vi "Demo.vi"() -> ()   [LabVIEW 2017]
uses:
  Components/ViPER.lvlibp/ViPER.lvclass
panel:
  in  "stop":bool
  out "error out":errorcluster
  in  "Config XML":string="<?xml version=\"1.0\" encoding=\"UTF-8\" standalone=\"no\" ?>\n<Object>\n\n  <Name>panel</Name>\n\n  <Class>DUT_Handler_Bailey_Panel</Class>\n\n  <Config>\n    <NumElts>1</NumElts>\n    <U32>\n      <Name>DUT Quantity</Name>\n      <Val>6</Val>\n</U32>\n</Config>  <Objects>\n    <Object>\n      <Name>Barcode</Name>\n      <Class>QR_Reader_Honeywell_3310G</Class>\n      <Config>\n        <NumElts>1</NumElts>\n        <Refnum>\n          <Name>ComPort</Name>\n          <RefKind>VISA</RefKind>\n          <Val>COM6</Val>\n</Refnum>\n</Config>    </Object>\n  </Objects>\n\n</Object>\n"
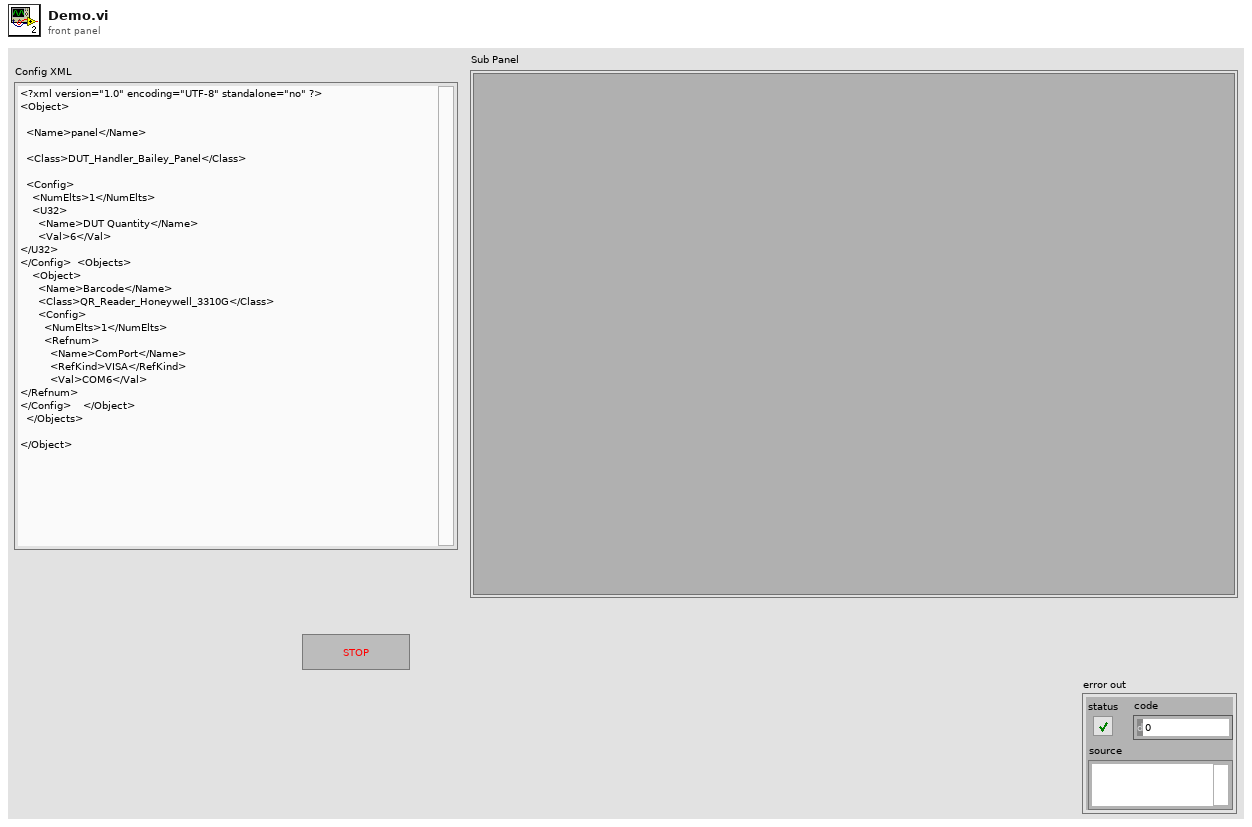
[diagram p1: front panel]
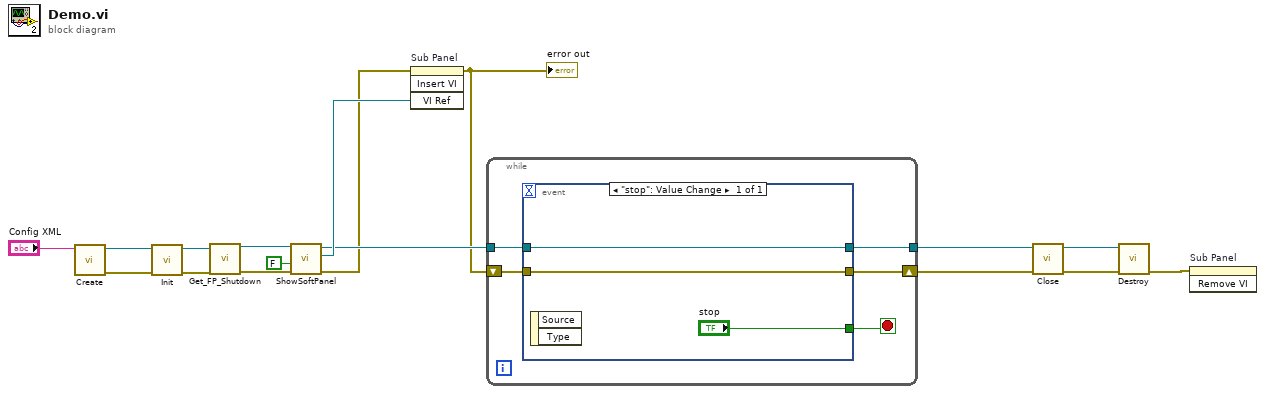
[diagram p0: block diagram]
diagram:
  n1 = call "Create.vi"("Config XML"="Config XML") -> ("error out"=w17:errorcluster, "reference out"=w16:refnum<class "ViPER.lvclass">)  [unwired: 9 in]
  n2 = call-dynamic "Init.vi"("error in (no error)"=w17, "reference in"=w16) -> ("error out"=w14:errorcluster, "reference out"=w13:refnum<class "ViPER.lvclass">)  [unwired: 8 in]
  n3 = call "Get_FP_Shutdown.vi"("ViKing_Base in"=w13, "error in (no error)"=w14) -> ("ViKing_Base out"=w11:refnum<class "ViPER.lvclass">, "error out"=w12:errorcluster)  [unwired: 9 in, 3 out]
  n4 = call-dynamic "ShowSoftPanel.vi"("error in (no error)"=w12, "Floating"=FALSE, "Driver in"=w11) -> ("error out"=w2:errorcluster, "vi reference"=w8:refnum<vi>, "Driver out"=w7:refnum<class "ViPER.lvclass">)  [unwired: 6 in]
  n5 = invoke on="Sub Panel" class="SubPnl" method="Insert VI"(error in=w2, "VI Ref"=w8) -> (error out=w1:errorcluster)  [unwired: 2 in, 3 out]
  "error out" <- w1
  n6 = while {
    tunnel: w7 -> [w21]
    shift-right: [w19] -> w5
    shift-left: w1 -> [w22]
    tunnel: [w18] -> w6
    stop <- w20 stop-if-true
    n7 = event shown="[0] \"stop\": Value Change" {
      selector: _ -> [_]
      dyn-events: _ -> [_]
      timeout: _ -> [_]
      tunnel: w22 -> [w24]
      tunnel: w21 -> [w23]
      tunnel: ["stop"] -> w20
      tunnel: [w24] -> w19
      tunnel: [w23] -> w18
      event "stop": Value Change {
        n8 = event-data() -> ()  [unwired: 1 in, 2 out]
      }
    }
  }
  n9 = call-dynamic "Close.vi"("error in (no error)"=w5, "reference in"=w6) -> ("error out"=w10:errorcluster, "reference out"=w9:refnum<class "ViPER.lvclass">)  [unwired: 8 in]
  n10 = call "Destroy.vi"("error in (no error)"=w10, "reference in"=w9) -> ("error out"=w4:errorcluster)  [unwired: 9 in]
  n11 = invoke on="Sub Panel" class="SubPnl" method="Remove VI"(error in=w4) -> ()  [unwired: 2 in, 3 out]
